vi "_miopen.vi"(2 "错误输入（无错误）":errorcluster, 3 "name":string, 4 "port":u16=1234, 5 "ip":string="192.168.1.44") -> (0 "错误输出":errorcluster, 1 "VISA引用句柄输出":refnum<visa-resource-name>)   [LabVIEW 2017]
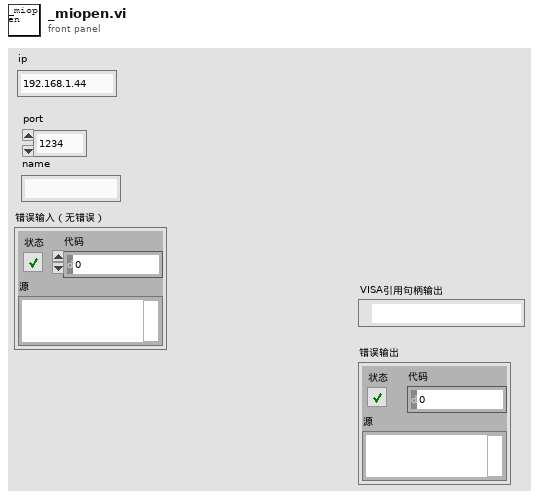
[diagram p1: front panel]
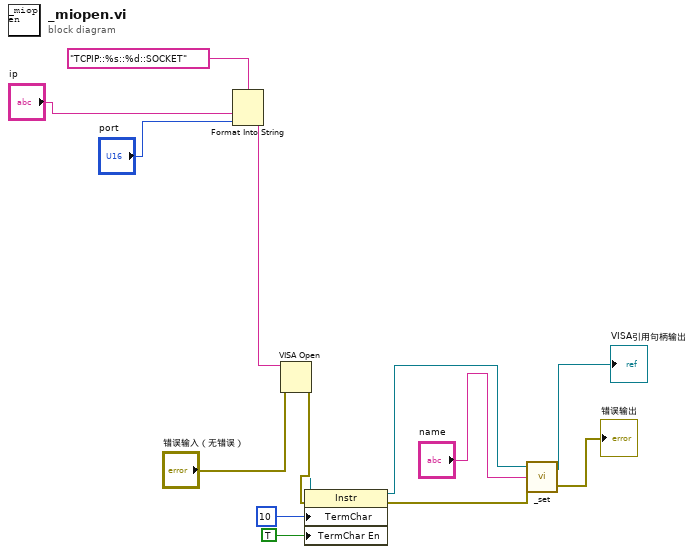
[diagram p0: block diagram]
diagram:
  n1 = Format Into String(format string="TCPIP::%s::%d::SOCKET" ("格式字符串"), "ip", "port") -> (resulting string=w1:string)  [unwired: 2 in, 1 out]
  n2 = VISA Open(error in (no error)="错误输入（无错误）", VISA resource name=w1) -> (VISA resource name=w11:refnum<visa-resource-name>, error out=w14:errorcluster)  [unwired: 3 in]
  n3 = property class="Instr"(reference=w11, error in=w14, "TermChar"=u8 10 ("Message Based Settings:Termination Character"), "TermChar En"=TRUE ("Message Based Settings:Termination Character Enable")) -> (reference out=w10:refnum<visa-resource-name>, error out=w8:errorcluster)
  n4 = call "_set.vi"("错误输入（无错误）"=w8, "写入缓冲区"="name", "VISA资源名称输出 2"=w10) -> ("错误输出"=→"错误输出":errorcluster, "VISA资源名称输出"=→"VISA引用句柄输出":refnum<visa-resource-name>)
